vi "Configure Output Channel Delay.vi"(7 "Output Off Delay Time (0 sec)":dbl, 8 "error in (no error)":errorcluster, 9 "Output On Delay Time (0 sec)":dbl, 10 "Channel (1)":string="1", 11 "VISA resource name":refnum<visa-resource-name>) -> (0 "error out":errorcluster, 3 "VISA resource name out":refnum<visa-resource-name>)   [LabVIEW 2020, in "Keysight E36300 Series.lvlib"]
doc: "Configures the delay in seconds that the power supply waits before enabling or disabling the specified output."
uses:
  Keysight E36300 Series.lvlib
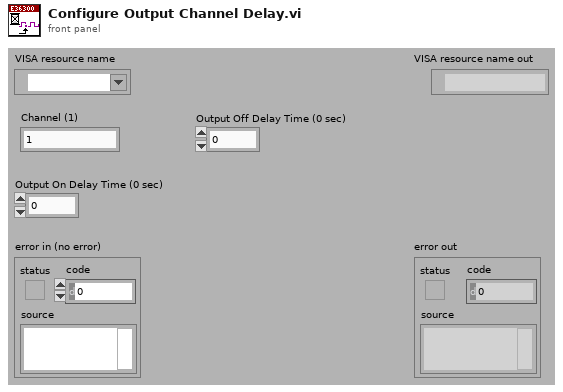
[diagram p1: front panel]
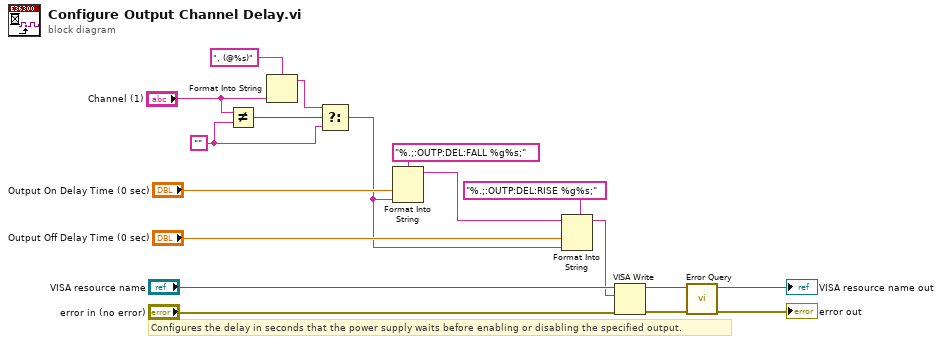
[diagram p0: block diagram]
diagram:
  w1 = ""
  # "Configures the delay in seconds that the power supply waits before enabling or disabling the specified output."
  n1 = Not Equal?(x="Channel (1)", y=w1) -> (x != y?=w4:bool)
  n2 = Format Into String(format string=", (@%s)", "Channel (1)") -> (resulting string=w5:string)  [unwired: 2 in, 1 out]
  n3 = Select(t=w5, s=w4, f=w1) -> (s? t:f=w2:string)
  n4 = Format Into String(format string="%.;:OUTP:DEL:FALL %g%s;", "Output On Delay Time (0 sec)", w2) -> (resulting string=w12:string)  [unwired: 2 in, 1 out]
  n5 = Format Into String(format string="%.;:OUTP:DEL:RISE %g%s;", initial string=w12, "Output Off Delay Time (0 sec)", w2) -> (resulting string=w8:string)  [unwired: 1 in, 1 out]
  n6 = VISA Write(VISA resource name="VISA resource name", write buffer=w8, error in (no error)="error in (no error)") -> (VISA resource name out=w16:refnum<visa-resource-name>, error out=w15:errorcluster)  [unwired: 1 out]
  n7 = call "Error Query.vi"("error in (no error)"=w15, "VISA resource name"=w16) -> ("error out"=→"error out":errorcluster, "VISA resource name out"=→"VISA resource name out":refnum<visa-resource-name>)  [unwired: 6 in, 2 out]
